vi "botones.vi"() -> ()   [LabVIEW 2020]
panel:
  out "Boton 6":bool
  out "Boton 5":bool
  out "Boton 4":bool
  out "Boton 3":bool
  out "Boton 2":bool
  out "Boton 1":bool
  in  "boton 6":bool
  in  "boton 5":bool
  in  "boton 4":bool
  in  "boton 3":bool
  in  "boton 2":bool
  in  "boton 1":bool
  # "Hasta dejar de presionar"
  # "El cambio solo ocurre\nunos instantes despues \nde ser presionado"
  # "Cambia de estado\ncuando presionas"
  # "Cambia de estado \ncuando sueltas el botón"
  # "Cambia de estado \ncuando sueltas"
  # "El cambio solo ocurre\nunos instantes despues \nde ser liberado"
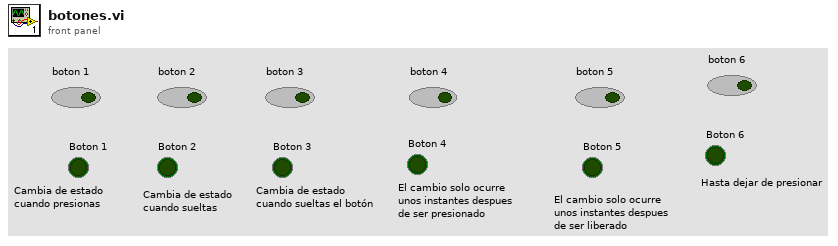
[diagram p1: front panel]
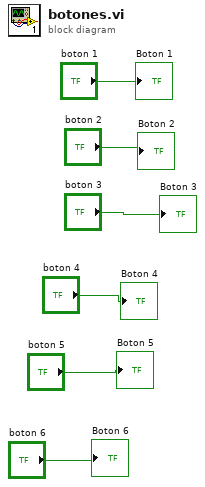
[diagram p0: block diagram]
diagram:
  "Boton 1" <- "boton 1"
  "Boton 2" <- "boton 2"
  "Boton 3" <- "boton 3"
  "Boton 4" <- "boton 4"
  "Boton 5" <- "boton 5"
  "Boton 6" <- "boton 6"
